vi "Initialize.vi"(8 "error in (no error)":errorcluster, 11 "JsonReportPlugin in":refnum<class "JsonReportPlugin.lvclass">) -> (0 "error out":errorcluster, 3 "JsonReportPlugin out":refnum<class "JsonReportPlugin.lvclass">)   [LabVIEW 2015, in "JsonReportPlugin.lvclass"]
uses:
  JsonReportPlugin.lvclass
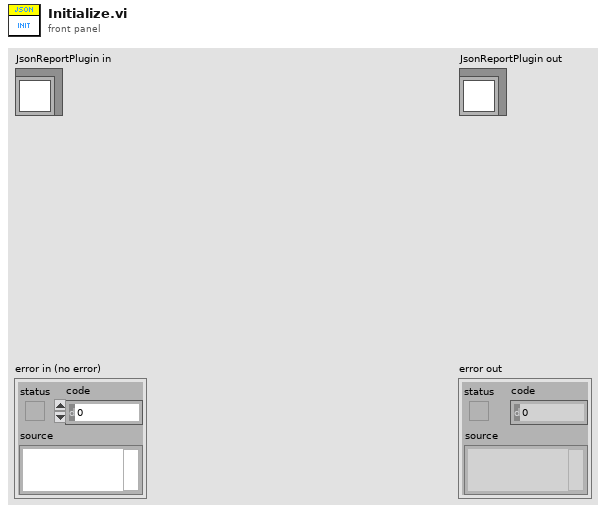
[diagram p1: front panel]
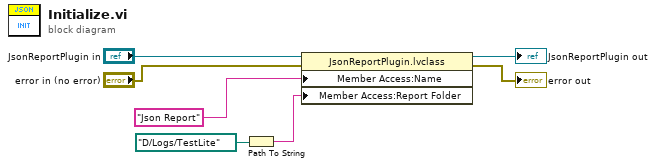
[diagram p0: block diagram]
diagram:
  n1 = Path To String(path=path "D:/Logs/TestLite" ("Report Folder")) -> (string=w1:string)
  n2 = property class="JsonReportPlugin.lvclass"(reference="JsonReportPlugin in", error in="error in (no error)", "Member Access:Name"="Json Report", "Member Access:Report Folder"=w1) -> (reference out=→"JsonReportPlugin out":refnum<class "JsonReportPlugin.lvclass">, error out=→"error out":errorcluster)
